vi "Imaging Data Display.vi"(0 "Frame number":i32, 9 "Filter gain":fxp<+,16,0>=0.8000030517578125, 11 "Kalman gain":fxp<+,16,1>=0.1015625) -> (4 "Image averaging done?":bool, 6 "Averaged image displayed?":bool, 8 "Frame imaging data Averaged?":bool, 10 "Averaged data address":u32, 14 "loop count":i32, 15 "Display_frames done":i32)   [LabVIEW 2015]
uses:
  <vilib>/Platform/TimedLoop/XDataNode/timing_clust.ctl
  <vilib>/Platform/TimedLoop/XDataNode/nitl_modes.ctl
  <vilib>/Platform/TimedLoop/XDataNode/wakeup.ctl
  OpenScan Labview code_20170126/DRAM data index.ctl
  <vilib>/rvi/Emulation/niFpgaGetClockAttributes.vi
  <vilib>/rvi/Emulation/niFpgaSctlEmulationGetInTimedLoop.vi
  <vilib>/rvi/Emulation/niFpgaEmulationReportErrorSimple.vi
  OpenScan Labview code_20170126/Global_Sample per Frame.vi
  <vilib>/rvi/Emulation/niFpgaCriticalErrorInLSC.vi
  <vilib>/rvi/DataTransferAndStorage/Container/Common/niFpgaContainerGetUniqueNameForEmu.vi
  <vilib>/rvi/DataTransferAndStorage/Container/Common/niFpgaContainerSetEmuInfo.vi
  <vilib>/rvi/eio/common/nirviEmuReportErrorAndStop.vi
  <vilib>/rvi/DataTransferAndStorage/Container/Common/niFpgaContainerExecOnDevCompGetState.vi
  <vilib>/rvi/Emulation/niFpgaEmulationIsFPGAContextNoSignature.vi
  <vilib>/rvi/errors/niFpgaSetErrorForExecOnDevCompSimple.vi
  <vilib>/rvi/FIFO/Fifo_Resource/nirvififoEmulationSetSize.vi
  <vilib>/rvi/FIFO/Fifo_Resource/nirviFifoEmulationQueueMgr.vi
  <instcachedir>/0/nirviFifoEmulationQueueMgr_E5CAEC123FF24DC58D834DCA3CDAA9B5.lvgen/nirviFifoEmulationQueueMgr_E5CAEC123FF24DC58D834DCA3CDAA9B5_002.vi
  <vilib>/rvi/FIFO/Fifo_Resource/nirvififoEmulationDetermineInputValidOut.vi
  <vilib>/rvi/FIFO/Fifo_Resource/nirvififoEmulationCreateLock.vi
  <vilib>/rvi/Emulation/niFpgaProcessEmulError.vi
  <vilib>/rvi/FIFO/Fifo_Resource/nirvififoEmulationObtainLock.vi
  <vilib>/rvi/FIFO/Fifo_Resource/nirvififoEmulationReleaseLock.vi
  <vilib>/rvi/occurrence/nirviWaitOnOccurrenceBase.vi
  <vilib>/rvi/errors/nirviReportUnexpectedCaseInternalError.vi
  <vilib>/rvi/errors/nirviReportUnexpectedCaseInternalError (U32).vi
  <vilib>/Utility/error.llb/Clear Errors.vi
  <vilib>/rvi/interface/RandomDataEmulation/niFpgaRandomDataHandleErrors.vi
  <vilib>/rvi/Memory/Memory_Emulation/niFpgaMemoryFastEmulationDramWriteAndRequestData.vi
  <vilib>/rvi/Memory/Memory_Emulation/niFpgaMemoryEmulationDramWriteAndRequestData.vi
  <vilib>/rvi/Memory/Memory_Emulation/niFpgaMemoryEmulationDramWriteAndRequestDataApplyByteEnables.vi
  <vilib>/rvi/LocalResourceManager/LocalResourceManager.xnode
  <vilib>/rvi/DataTransferAndStorage/Container/XNode/niFpgaContainer.xnode
  <vilib>/rvi/FIFO/Fifo_Resource/niFpgaFifoEmulationRefIn.vi
  <vilib>/Platform/TimedLoop/XDataNode/XDataNode.xnode
  <vilib>/rvi/Memory/Memory_Emulation/niFpgaMemoryEmulationDramRetrieveData.vi
  <vilib>/rvi/FIFO/Fifo_Resource/nirvififoEmulationWrite.vi
  <vilib>/rvi/FIFO/Fifo_Resource/nirvififoEmulationRead.vi
  <vilib>/rvi/interface/RandomDataEmulation/nirviRandomDataFpgaReadWriteTemplate.vi
  <vilib>/Platform/TimedLoop/XDataNode/XDNodeRunTimeDep.lvlib
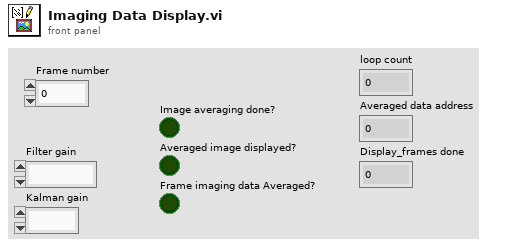
[diagram p1: front panel]
types:
  T1 = cluster{"Numeric 1":u32, "Numeric 2":u32, "Numeric 3":u32, "Numeric 4":u32, "Numeric 5":u32, "Numeric 6":u32, "Numeric 7":u32, "Numeric 8":u32, "Numeric 9":u32, "Numeric 10":u32, "Numeric 11":u32, "Numeric 12":u32, "Numeric 13":u32, "Numeric 14":u32, "Numeric 15":u32, "Numeric 16":u32}
  T2 = typedef "DRAM data index.ctl" = enum16{"Numeric 1", "Numeric 2", "Numeric 3", "Numeric 4", "Numeric 5", "Numeric 6", "Numeric 7", "Numeric 8", "Numeric 9", "Numeric 10", "Numeric 11", "Numeric 12", "Numeric 13", "Numeric 14", "Numeric 15", "Numeric 16"}
  T3 = typedef "XDNodeRunTimeDep.lvlib/timing_clust.ctl" = cluster{"Expected End [f-1]":u64, "Actual End [f-1]":u64, "Finished Late? [f-1]":bool, "Expected End [i-1]":u64, "Actual End [i-1]":u64, "Finished Late? [i-1]":bool, "Expected Start [i]":u64, "Actual Start [i]":u64, "Expected Start [f]":u64, "Actual Start [f]":u64, "Source Name":string, "Structure Name":string, "Period":i64, "Deadline":i64, "Offset":i64, "Start":i64, "Priority":i32, "Timeout":i32, "Mode":T4, "Wakeup Reason":T5, "Error":errorcluster, "Source Type":string, "Secondary Source Type":string, "Global End Time":u64, "Global Start Time":u64, "Frame Duration":u64, "Iteration Duration":u64, "Assigned CPU":i32, "I/O Scan Engine Mode":u32}
  T4 = typedef "XDNodeRunTimeDep.lvlib/nitl_modes.ctl" = enum32{"No Change", "Process missed periods, maintain original phase", "Discard missed periods, maintain original phase", "Process missed periods, ignore original phase", "Discard missed periods, ignore original phase"}
  T5 = typedef "XDNodeRunTimeDep.lvlib/wakeup.ctl" = enum32{"Normal", "Aborted", "Asynchronous wakeup", "Timing source error", "Timed loop error", "Timeout"}
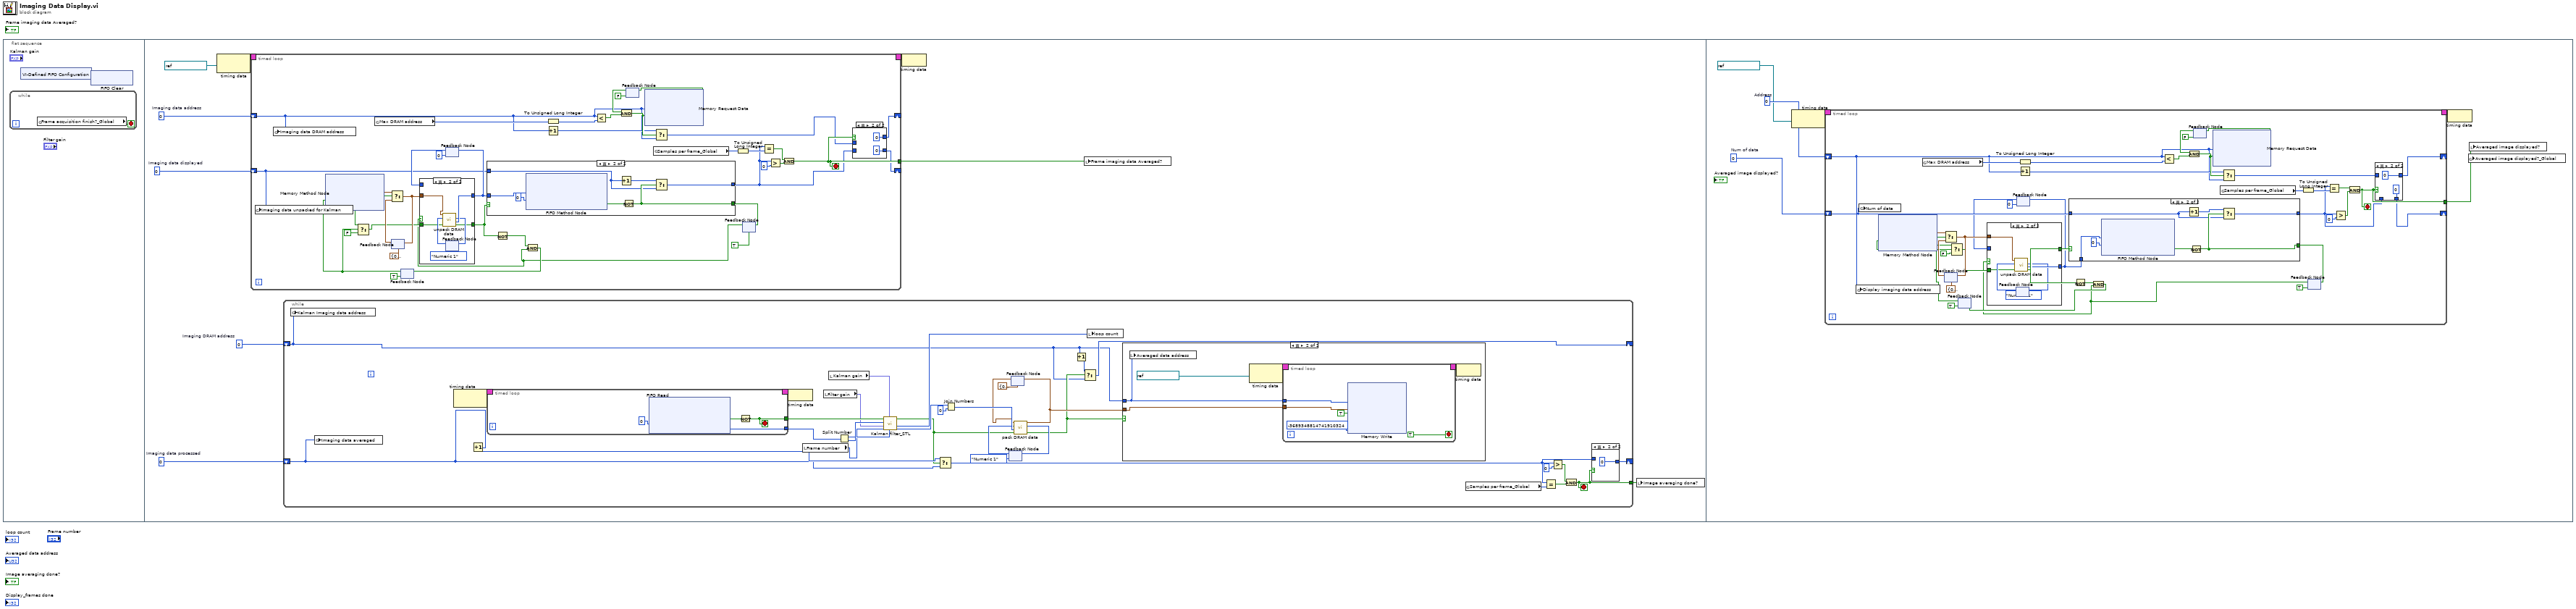
[diagram p0: block diagram]
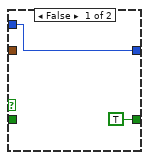
[diagram p4: hidden frame]
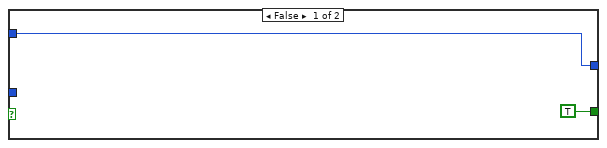
[diagram p6: hidden frame]
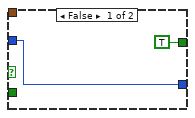
[diagram p7: hidden frame]
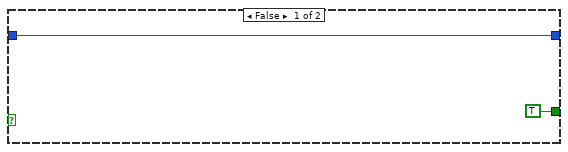
[diagram p9: hidden frame]
diagram:
  n1 = flat-sequence {
    frame #0 {
      n2 = while {
        stop <- w2 stop-if-true
        n3 = global read "Global_Sample per Frame.vi" "Frame acquisition finish?_Global"() -> (w2:bool)
      }
      n4 = xnode "VI-Defined FIFO Configuration"() -> ("FIFO输出"=w1:refnum<k21>)
      n5 = xnode ("FIFO Clear")("FIFO输入"=w1) -> ()  [unwired: 1 out]
    }
    frame #1 {
      w3 = u32 0  # Imaging DRAM address
      w6 = u32 0  # Imaging data processed
      w8 = u32 0  # Imaging data displayed
      w9 = u32 0  # Imaging data address
      n6 = node-c288(refnum<k21> "DRAM Clock" ("Source Name")) -> (w11:T3)
      n7 = timed-loop {
        shift-right: [w88] -> _
        shift-left: w9 -> [w74]
        timing: w11 -> [_]
        timing-out: [_] -> w10
        shift-right: [w87] -> _
        shift-left: w8 -> [w73]
        tunnel: [w91] -> w5
        stop <- w91 stop-if-true
        n8 = global write "Global_Sample per Frame.vi" "Imaging data unpacked for Kalman"(w73) -> ()
        n9 = global write "Global_Sample per Frame.vi" "Imaging data DRAM address"(w74) -> ()
        n10 = global read "Global_Sample per Frame.vi" "Max DRAM address"() -> (w93:u32)
        n11 = feedback #1(T1 {"Numeric 1"=0, "Numeric 2"=0, "Numeric 3"=0, "Numeric 4"=0, "Numeric 5"=0, "Numeric 6"=0, "Numeric 7"=0, "Numeric 8"=0, "Numeric 9"=0, "Numeric 10"=0, "Numeric 11"=0, "Numeric 12"=0, "Numeric 13"=0, "Numeric 14"=0, "Numeric 15"=0, "Numeric 16"=0} ("Data")) -> (w100:T1)
        n12 = feedback #2(TRUE) -> (w81:bool)
        n13 = xnode ("Memory Method Node")("输出就绪"=w81) -> ("数据"=w103:T1, "输出有效"=w80:bool)  [unwired: 1 in, 1 out]
        n14 = Select(t=w80, s=w81, f=FALSE) -> (s? t:f=w78:bool)
        n15 = Select(t=w103, s=w80, f=w100) -> (s? t:f=w86:T1)
        n16 = feedback-in #1(w86) -> ()
        n17 = feedback #3(u32 0 ("Unpacked data")) -> (w76:u32)
        n18 = To Unsigned Long Integer(number=w93) -> (unsigned 32bit integer=w99:u32)
        n19 = Increment(x=w74) -> (x+1=w104:u32)
        n20 = Less?(x=w74, y=w99) -> (x < y?=w108:bool)
        n21 = feedback #4(FALSE ("Ready for Input")) -> (w106:bool)
        n22 = And(x=w106, y=w108) -> (x .and. y?=w105:bool)
        n23 = xnode ("Memory Request Data")("地址"=w74, "输入有效"=w105) -> ("输入就绪"=w107:bool)  [unwired: 1 in, 1 out]
        n24 = feedback-in #4(w107) -> ()
        n25 = global read "Global_Sample per Frame.vi" "Samples per frame_Global"() -> (w92:u32)
        n26 = Select(t=w104, s=w105, f=w74) -> (s? t:f=w90:u32)
        n27 = To Unsigned Long Integer(number=w92) -> (unsigned 32bit integer=w98:u32)
        n28 = feedback #5(TRUE) -> (w77:bool)
        n29 = case shown="真" w77 {
          tunnel: w86 -> [_ w117]
          tunnel: [w110 w116] -> w75
          tunnel: [TRUE ("output valid?") w112] -> w85
          tunnel: w78 -> [_ w111]
          tunnel: w76 -> [w110 _]
          frame False {
          }
          frame True {
            n30 = feedback #6(DRAM_data_index."Numeric 1" ("DRAM pack index out")) -> (w114:T2)
            n31 = call "unpack DRAM data.vi"("input valid?"=w111, "DRAM pack index in"=w114, "packer in"=w117) -> ("output valid?"=w112:bool, "Unpacked data"=w116:u32, "DRAM pack index out"=w115:T2)  [unwired: 5 in, 1 out]
            n32 = feedback-in #6(w115) -> ()
          }
        }
        n33 = feedback-in #3(w75) -> ()
        n34 = case shown="真" w85 {
          tunnel: [TRUE w127] -> w102
          tunnel: w75 -> [_ w124]
          tunnel: w73 -> [w122 w126]
          tunnel: [w122 w125] -> w89
          frame False {
          }
          frame True {
            n35 = xnode ("FIFO Method Node")("元素"=w124, "超时"=0 ("Timeout")) -> ("超时？"=w129:bool)  [unwired: 1 in, 1 out]
            n36 = Increment(x=w126) -> (x+1=w128:u32)
            n37 = Not(x=w129) -> (.not. x?=w127:bool)
            n38 = Select(t=w128, s=w127, f=w126) -> (s? t:f=w125:u32)
          }
        }
        n39 = Not(x=w85) -> (.not. x?=w84:bool)
        n40 = And(x=w84, y=w77) -> (x .and. y?=w83:bool)
        n41 = feedback-in #2(w83) -> ()
        n42 = feedback-in #5(w102) -> ()
        n43 = Equal?(x=w89, y=w98) -> (x = y?=w95:bool)
        n44 = Greater?(x=w89, y=u32 0) -> (0:w96:bool)
        n45 = And(x=w95, y=w96) -> (x .and. y?=w91:bool)
        n46 = case shown="真" w91 {
          tunnel: w90 -> [w118 _]
          tunnel: w89 -> [w119 _]
          tunnel: [w118 u32 0 ("Imaging data address")] -> w88
          tunnel: [w119 u32 0 ("Imaging data displayed")] -> w87
          frame False {
          }
          frame True {
          }
        }
      }
      n47 = while {
        shift-right: [w38] -> _
        shift-left: w6 -> [w14]
        tunnel: [w39] -> w4
        shift-right: [w16] -> _
        shift-left: w3 -> [w15]
        stop <- w39 stop-if-true
        n48 = global write "Global_Sample per Frame.vi" "Kalman Imaging data address"(w15) -> ()
        n49 = global write "Global_Sample per Frame.vi" "Imaging data averaged"(w14) -> ()
        n50 = node-c288() -> (w13:T3)  [unwired: 1 in]
        n51 = Increment(x=w14) -> (x+1=w31:u32)
        n52 = timed-loop {
          tunnel: [w45] -> w44
          tunnel: [w46] -> w36
          timing: w13 -> [_]
          timing-out: [_] -> w12
          stop <- w45 stop-if-true
          n53 = xnode ("FIFO Read")("超时"=0 ("Timeout")) -> ("元素"=w46:u32, "超时？"=w47:bool)  [unwired: 1 in, 1 out]
          n54 = Not(x=w47) -> (.not. x?=w45:bool)
        }
        n55 = node-c288(w12) -> ()
        n56 = local read "Frame number"() -> (w27:i32)
        n57 = local read "Filter gain"() -> (w29:fxp<+,16,0>)
        n58 = local read "Kalman gain"() -> (w30:fxp<+,16,1>)
        n59 = Split Number(x=w36) -> (hi(x)=w34:u16, lo(x)=w35:u16)
        n60 = call "Kalman filter_STL.vi"("Previous predicted pixel value"=w34, "Kalman gain"=w30, "Frame number"=w27, "Filter gain"=w29, "Pixel value"=w35, "Input valid"=w44) -> ("Kalman filter result"=w33:u16, "loop count"=w28:i32, "output valid"=w22:bool)  [unwired: 3 in]
        n61 = Select(t=w31, s=w22, f=w14) -> (s? t:f=w37:u32)
        n62 = Join Numbers(hi=w33, lo=u16 0) -> ((hi.lo)=w26:u32)
        n63 = feedback #7(DRAM_data_index."Numeric 1" ("DRAM Index out")) -> (w24:T2)
        n64 = feedback #8(T1 {"Numeric 1"=0, "Numeric 2"=0, "Numeric 3"=0, "Numeric 4"=0, "Numeric 5"=0, "Numeric 6"=0, "Numeric 7"=0, "Numeric 8"=0, "Numeric 9"=0, "Numeric 10"=0, "Numeric 11"=0, "Numeric 12"=0, "Numeric 13"=0, "Numeric 14"=0, "Numeric 15"=0, "Numeric 16"=0} ("packer out")) -> (w21:T1)
        n65 = call "pack DRAM data.vi"("input valid?"=w22, "data to be packed"=w26, "DRAM Index in"=w24, "packer in"=w21) -> ("output valid?"=w18:bool, "DRAM Index out"=w25:T2, "packer out"=w20:T1)  [unwired: 5 in]
        n66 = feedback-in #7(w25) -> ()
        n67 = feedback-in #8(w20) -> ()
        n68 = Increment(x=w15) -> (x+1=w17:u32)
        n69 = Select(t=w17, s=w18, f=w15) -> (s? t:f=w16:u32)
        n70 = local write "loop count"(w28) -> ()
        n71 = case shown="真" w18 {
          tunnel: w15 -> [_ w54]
          tunnel: w20 -> [_ w53]
          frame False {
          }
          frame True {
            n72 = local write "Averaged data address"(w54) -> ()
            n73 = node-c288(refnum<k21> "DRAM Clock" ("Source Name")) -> (w57:T3)
            n74 = timed-loop {
              timing: w57 -> [_]
              timing-out: [_] -> w56
              tunnel: w54 -> [w62]
              tunnel: w53 -> [w58]
              stop <- TRUE stop-if-true
              n75 = xnode ("Memory Write")("地址"=w62, "数据"=w58, "输入有效"=TRUE ("Input Valid"), "字节启用"=i64 -3689348814741910324 ("Byte Enables")) -> ()  [unwired: 1 in, 2 out]
            }
            n76 = node-c288(w56) -> ()
          }
        }
        n77 = global read "Global_Sample per Frame.vi" "Samples per frame_Global"() -> (w40:u32)
        n78 = Equal?(x=w37, y=w40) -> (x = y?=w41:bool)
        n79 = Greater?(x=w37, y=u32 0) -> (0:w42:bool)
        n80 = And(x=w42, y=w41) -> (x .and. y?=w39:bool)
        n81 = case shown="真" w39 {
          tunnel: [w69 u32 0 ("Imaging data address")] -> w38
          tunnel: w37 -> [w69 _]
          frame False {
          }
          frame True {
          }
        }
      }
      n82 = node-c288(w10) -> ()
      n83 = local write "Frame imaging data Averaged?"(w5) -> ()
      n84 = local write "Image averaging done?"(w4) -> ()
    }
    frame #2 {
      w139 = u32 0  # Address
      w140 = u32 0  # Num of data
      n85 = node-c288(refnum<k21> "DRAM Clock" ("Source Name")) -> (w142:T3)
      n86 = timed-loop {
        shift-right: [w158] -> _
        shift-left: w139 -> [w161]
        timing: w142 -> [_]
        timing-out: [_] -> w141
        shift-right: [w155] -> _
        shift-left: w140 -> [w160]
        tunnel: [w157] -> w137
        stop <- w157 stop-if-true
        n87 = global write "Global_Sample per Frame.vi" "Display imaging data address"(w161) -> ()
        n88 = global write "Global_Sample per Frame.vi" "Num of data"(w160) -> ()
        n89 = global read "Global_Sample per Frame.vi" "Max DRAM address"() -> (w163:u32)
        n90 = feedback #9(T1 {"Numeric 1"=0, "Numeric 2"=0, "Numeric 3"=0, "Numeric 4"=0, "Numeric 5"=0, "Numeric 6"=0, "Numeric 7"=0, "Numeric 8"=0, "Numeric 9"=0, "Numeric 10"=0, "Numeric 11"=0, "Numeric 12"=0, "Numeric 13"=0, "Numeric 14"=0, "Numeric 15"=0, "Numeric 16"=0} ("Data")) -> (w172:T1)
        n91 = feedback #10(TRUE) -> (w149:bool)
        n92 = xnode ("Memory Method Node")("输出就绪"=w149) -> ("数据"=w175:T1, "输出有效"=w170:bool)  [unwired: 1 in, 1 out]
        n93 = Select(t=w175, s=w149, f=w172) -> (s? t:f=w154:T1)
        n94 = feedback-in #9(w154) -> ()
        n95 = Select(t=w170, s=w149, f=FALSE) -> (s? t:f=w153:bool)
        n96 = feedback #11(u32 0 ("Unpacked data")) -> (w146:u32)
        n97 = To Unsigned Long Integer(number=w163) -> (unsigned 32bit integer=w169:u32)
        n98 = Increment(x=w161) -> (x+1=w176:u32)
        n99 = Less?(x=w161, y=w169) -> (x < y?=w180:bool)
        n100 = feedback #12(FALSE ("Ready for Input")) -> (w178:bool)
        n101 = And(x=w178, y=w180) -> (x .and. y?=w177:bool)
        n102 = xnode ("Memory Request Data")("地址"=w161, "输入有效"=w177) -> ("输入就绪"=w179:bool)  [unwired: 1 in, 1 out]
        n103 = feedback-in #12(w179) -> ()
        n104 = global read "Global_Sample per Frame.vi" "Samples per frame_Global"() -> (w162:u32)
        n105 = Select(t=w176, s=w177, f=w161) -> (s? t:f=w159:u32)
        n106 = To Unsigned Long Integer(number=w162) -> (unsigned 32bit integer=w168:u32)
        n107 = feedback #13(TRUE) -> (w147:bool)
        n108 = case shown="真" w147 {
          tunnel: w154 -> [_ w189]
          tunnel: [w182 w188] -> w145
          tunnel: w153 -> [_ w184]
          tunnel: [TRUE ("output valid?") w183] -> w152
          tunnel: w146 -> [w182 _]
          frame False {
          }
          frame True {
            n109 = feedback #14(DRAM_data_index."Numeric 1" ("DRAM pack index out")) -> (w186:T2)
            n110 = call "unpack DRAM data.vi"("input valid?"=w184, "DRAM pack index in"=w186, "packer in"=w189) -> ("output valid?"=w183:bool, "Unpacked data"=w188:u32, "DRAM pack index out"=w187:T2)  [unwired: 5 in, 1 out]
            n111 = feedback-in #14(w187) -> ()
          }
        }
        n112 = feedback-in #11(w145) -> ()
        n113 = case shown="真" w152 {
          tunnel: [TRUE w199] -> w174
          tunnel: w160 -> [w194 w198]
          tunnel: [w194 w197] -> w156
          tunnel: w145 -> [_ w196]
          frame False {
          }
          frame True {
            n114 = xnode ("FIFO Method Node")("元素"=w196, "超时"=0 ("Timeout")) -> ("超时？"=w201:bool)  [unwired: 1 in, 1 out]
            n115 = Increment(x=w198) -> (x+1=w200:u32)
            n116 = Not(x=w201) -> (.not. x?=w199:bool)
            n117 = Select(t=w200, s=w199, f=w198) -> (s? t:f=w197:u32)
          }
        }
        n118 = Not(x=w152) -> (.not. x?=w151:bool)
        n119 = And(x=w151, y=w147) -> (x .and. y?=w150:bool)
        n120 = feedback-in #10(w150) -> ()
        n121 = feedback-in #13(w174) -> ()
        n122 = Equal?(x=w156, y=w168) -> (x = y?=w165:bool)
        n123 = Greater?(x=w156, y=u32 0) -> (0:w166:bool)
        n124 = And(x=w165, y=w166) -> (x .and. y?=w157:bool)
        n125 = case shown="真" w157 {
          tunnel: w159 -> [w191 _]
          tunnel: [w191 u32 0 ("Address")] -> w158
          tunnel: w156 -> [w190 _]
          tunnel: [w190 u32 0 ("Num of data")] -> w155
          frame False {
          }
          frame True {
          }
        }
      }
      n126 = node-c288(w141) -> ()
      n127 = global write "Global_Sample per Frame.vi" "Averaged image displayed?_Global"(w137) -> ()
      n128 = local write "Averaged image displayed?"(w137) -> ()
    }
  }
